vi "TestPointer.Allocate Empty Byte Array.vi"(8 "error in (no error)":errorcluster, 11 "Test Pointer in":refnum<class "TestPointer.lvclass">) -> (0 "error out":errorcluster, 2 "empty byte array":u8[](array[numeric]), 3 "Test Pointer out":refnum<class "TestPointer.lvclass">)   [LabVIEW 2016, in "TestPointer.lvclass"]
uses:
  TestPointer.lvclass
  C:/Git/LabVIEW-Memory/Source/Classes/Pointer/Pointer.lvclass
  Source/Classes/Pointer/Pointer.lvclass
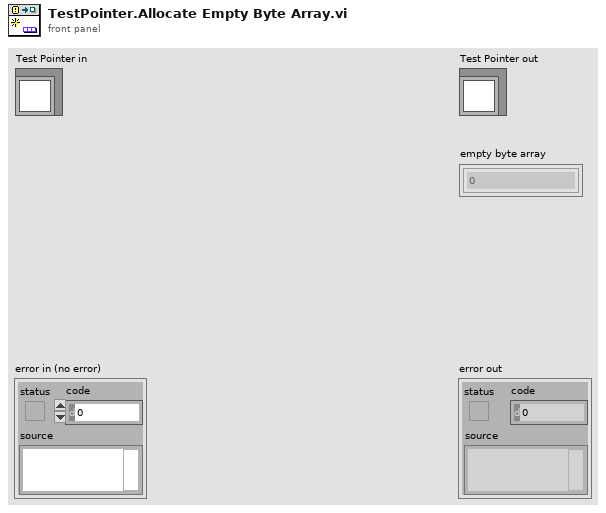
[diagram p1: front panel]
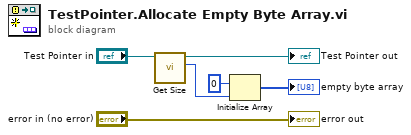
[diagram p0: block diagram]
diagram:
  n1 = call "Get Size.vi"("Pointer in"="Test Pointer in") -> ("size"=w6:u64, "Pointer out"=→"Test Pointer out":refnum<class "TestPointer.lvclass">)  [unwired: 9 in]
  n2 = Initialize Array(u8 0 ("element"), w6) -> (→"empty byte array":u8[])
  "error out" <- "error in (no error)"
